vi "Select User Message.vi"(8 "error in (no error)":errorcluster, 10 "Message Selector":T1, 11 "View Model":T3) -> (0 "error out":errorcluster, 1 "Message":string, 3 "View Model":T3)   [LabVIEW 2017]
doc: "Select User Message from List and replace Dynamic data.\n[Covers: UM1A]"
uses:
  View Model/Controls/View Model.ctl
  View Model/Controls/Shared Model.ctl
  Error Handler/Controls/Error Model.ctl
  Error Handler/Controls/Error Data.ctl
  Error Handler/Controls/Error Type.ctl
  Error Handler/Controls/Error Source.ctl
  Configuration/Controls/Config Model.ctl
  Configuration/Controls/Config CMD.ctl
  Configuration/Controls/Config Command.ctl
  Controls/Controller Model.ctl
  Controls/Controller Overhead.ctl
  Controls/Controller Transaction.ctl
  Controls/Controller State.ctl
  Configuration/Controls/Config Data Record.ctl
  Controls/Controller Message Selector.ctl
  Controls/Controller Message Type.ctl
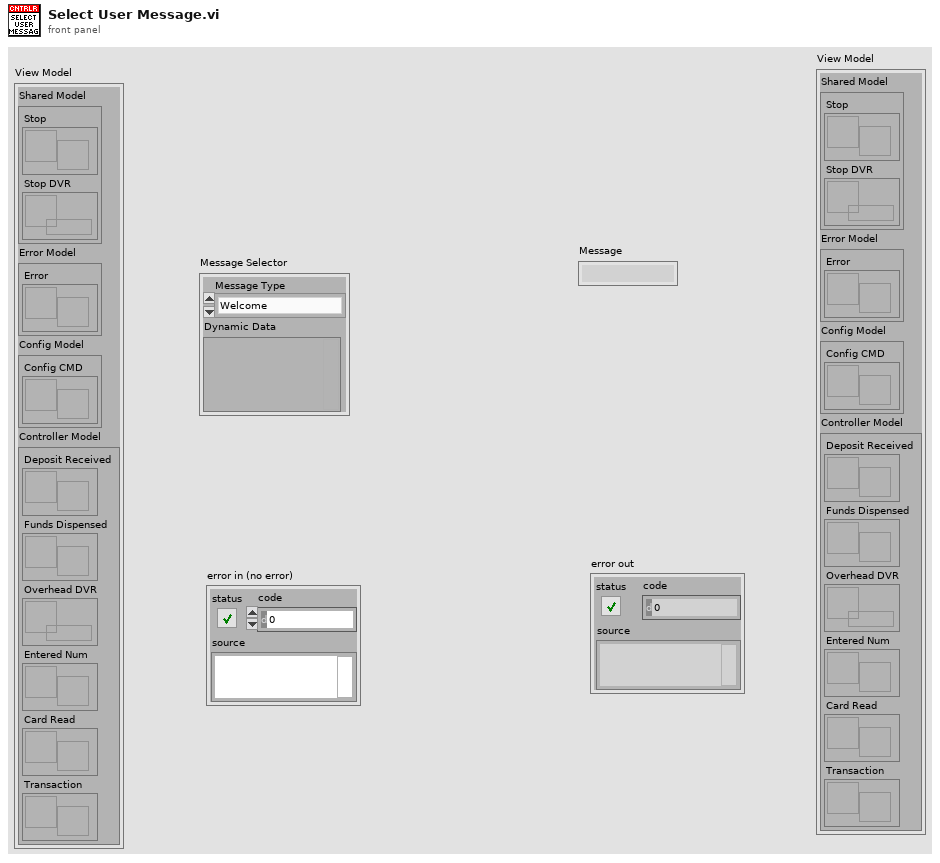
[diagram p1: front panel]
types:
  T1 = typedef "Controller Message Selector.ctl" = cluster{"Message Type":T2, "Dynamic Data":variant}
  T2 = typedef "Controller Message Type.ctl" = enum16{"Welcome", "Login", "Idle", "Invalid Login", "Terminate Session", "Deposit", "Withdrawal", "Fast Cash", "Withdrawal Complete", "Withdrawal Failed", "Balance"}
  T3 = typedef "View Model.ctl" = cluster{"Shared Model":T4, "Error Model":T5, "Config Model":T6, "Controller Model":T7}
  T4 = typedef "Shared Model.ctl" = cluster{"Stop":refnum<user-event>, "Stop DVR":refnum<data-value>}
  T5 = typedef "Error Model.ctl" = cluster{"Error":refnum<user-event>}
  T6 = typedef "Config Model.ctl" = cluster{"Config CMD":refnum<user-event>}
  T7 = typedef "Controller Model.ctl" = cluster{"Deposit Received":refnum<user-event>, "Funds Dispensed":refnum<user-event>, "Overhead DVR":refnum<data-value>, "Entered Num":refnum<user-event>, "Card Read":refnum<user-event>, "Transaction":refnum<user-event>}
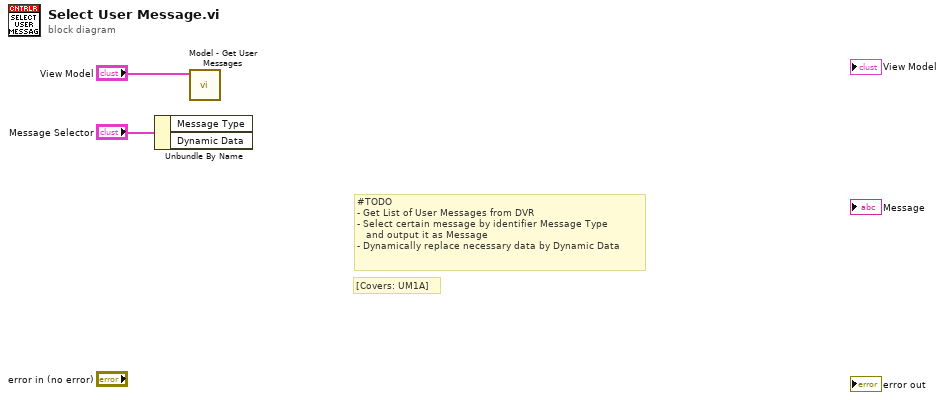
[diagram p0: block diagram]
diagram:
  # "[Covers: UM1A]"
  # "#TODO\n- Get List of User Messages from DVR\n- Select certain message by identifier Message Type\n   and output it as Message\n- Dynamically replace necessary data by Dynamic Data"
  n1 = Unbundle By Name("Message Selector") -> ()  [unwired: 2 out]
  n2 = call "Model - Get User Messages.vi"("View Model"="View Model") -> ()  [unwired: 8 in, 3 out]
